vi "SwerveUnwrapGoalAngle.vi"(1 "Current Unwrapped Angle (deg) [-Inf,+Inf]":dbl, 2 "Flipped Goal Angle (deg) [-180, +180]":dbl) -> (0 "Absolute Azimuth Position (tics) [-Inf,+Inf]":dbl)   [LabVIEW 2020]
doc: "Unwraps the goal azimuth angle from [-180,+180] to [-Inf,+Inf] and converts it to tics so that the control loop can run directly on the azimuth Falcon."
uses:
  GlobalDrivebase.vi
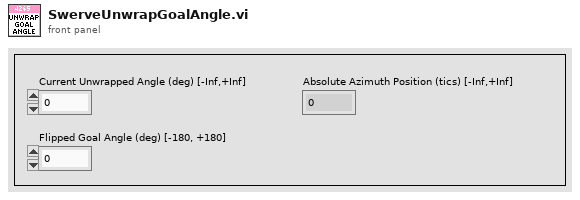
[diagram p1: front panel]
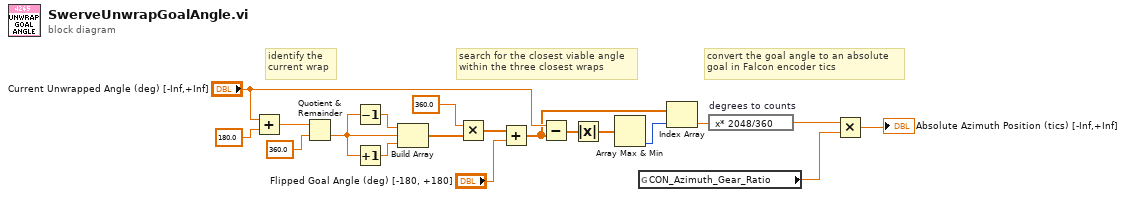
[diagram p0: block diagram]
diagram:
  # "convert the goal angle to an absolute\ngoal in Falcon encoder tics"
  # "search for the closest viable angle\nwithin the three closest wraps"
  # "identify the\ncurrent wrap"
  n1 = Add(x="Current Unwrapped Angle (deg) [-Inf,+Inf]", y=180.0) -> (x+y=w6:dbl)
  n2 = Quotient & Remainder(x=w6, y=360.0) -> (floor(x/y)=w10:dbl)  [unwired: 1 out]
  n3 = Decrement(x=w10) -> (x-1=w9:dbl)
  n4 = Increment(x=w10) -> (x+1=w11:dbl)
  n5 = Build Array(w9, w10, w11) -> (w18:dbl[])
  n6 = Multiply(x=360.0, y=w18) -> (x*y=w12:dbl[])
  n7 = Add(x=w12, y="Flipped Goal Angle (deg) [-180, +180]") -> (x+y=w4:dbl[])
  n8 = Subtract(x="Current Unwrapped Angle (deg) [-Inf,+Inf]", y=w4) -> (x-y=w15:dbl[])
  n9 = Absolute Value(x=w15) -> (abs(x)=w16:dbl[])
  n10 = Array Max & Min(array=w16) -> (min index (indices)=w17:i32)  [unwired: 3 out]
  n11 = global read "GlobalDrivebase.vi" "CON_Azimuth_Gear_Ratio"() -> (w1:dbl)
  n12 = Index Array(array=w4, index=w17) -> (element=w19:dbl)
  n13 = expression code="x* 2048/360" "degrees to counts"(w19) -> (w3:dbl)
  n14 = Multiply(x=w3, y=w1) -> (x*y=→"Absolute Azimuth Position (tics) [-Inf,+Inf]":dbl)
